vi "RankMinimalSchedule.vi"(8 "error in (no error)":errorcluster, 11 "OSSP_Problem in":refnum<class "OSSP_Problem.lvclass">) -> (0 "error out":errorcluster, 2 "Schedule Out":i32[](array[numeric]), 3 "OSSP_Problem out":refnum<class "OSSP_Problem.lvclass">)   [LabVIEW 2013, in "GA.lvclass"]
uses:
  GA.lvclass
  OSSP_Problem.lvclass
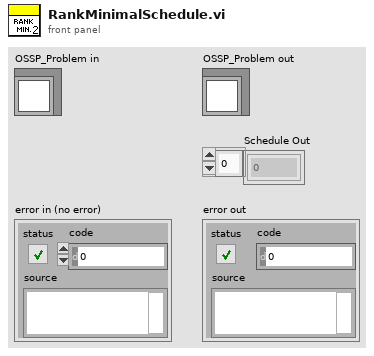
[diagram p1: front panel]
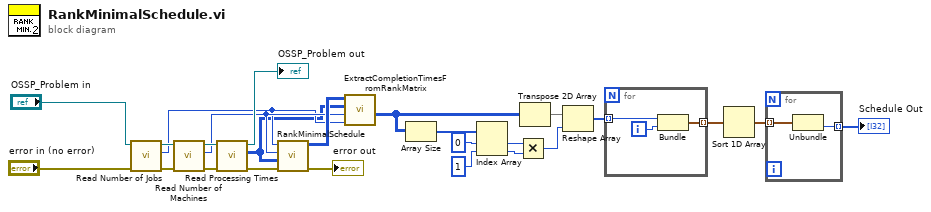
[diagram p0: block diagram]
diagram:
  n1 = call-dynamic "Read Number of Jobs.vi"("error in (no error)"="error in (no error)", "OSSP_Problem in"="OSSP_Problem in") -> ("error out"=w19:errorcluster, "Number of Jobs"=w5:i32, "OSSP_Problem out"=w20:refnum<class "OSSP_Problem.lvclass">)  [unwired: 7 in]
  n2 = call-dynamic "Read Number of Machines.vi"("error in (no error)"=w19, "OSSP_Problem in"=w20) -> ("error out"=w18:errorcluster, "Number of Machines"=w6:i32, "OSSP_Problem out"=w17:refnum<class "OSSP_Problem.lvclass">)  [unwired: 7 in]
  n3 = call-dynamic "Read Processing Times.vi"("error in (no error)"=w18, "OSSP_Problem in"=w17) -> ("error out"=w16:errorcluster, "Processing Times"=w1:u16[][], "OSSP_Problem out"=→"OSSP_Problem out":refnum<class "OSSP_Problem.lvclass">)  [unwired: 7 in]
  n4 = call "RankMinimalSchedule.vi"("error in (no error)"=w16, "Processing Time Matrix In"=w1, "Number of Machines"=w6, "NUmber Of Jobs"=w5) -> ("error out"=→"error out":errorcluster, "Rank Minimal Matrix"=w15:i32[][])  [unwired: 6 in]
  n5 = call "ExtractCompletionTimesFromRankMatrix.vi"("Number of  Jobs"=w5, "Number of Machines"=w6, "Processing Times"=w1, "Rank Matrix"=w15) -> ("Start Times"=w3:u16[][])  [unwired: 4 in, 3 out]
  n6 = Array Size(array=w3) -> (size(s)=w14:i32[])
  n7 = Index Array(array=w14, index #1=0 ("index"), index #2=1 ("index")) -> (element #1=w11:i32, element #2=w10:i32)
  n8 = Multiply(x=w11, y=w10) -> (x*y=w4:i32)
  n9 = Transpose 2D Array(2D array=w3) -> (transposed array=w2:u16[][])
  n10 = Reshape Array(w2, w4) -> (w9:u16[])
  n11 = for {
    tunnel: w9 -> [w28] mode=indexing
    tunnel: [w26] -> w8 mode=indexing
    i -> [w27]
    n12 = Bundle("element"=w28, w27) -> (w26:cluster{"element":u16, i32})  [unwired: 1 in]
  }
  n13 = Sort 1D Array(array=w8) -> (sorted array=w7:cluster{"element":u16, i32}[])
  n14 = for {
    tunnel: w7 -> [w30] mode=indexing
    tunnel: [w29] -> w25 mode=indexing
    n15 = Unbundle(w30) -> (w29:i32)  [unwired: 1 out]
  }
  "Schedule Out" <- w25
